vi "19.2-Signal-Generator-FFT.vi"() -> ()   [LabVIEW 2020]
uses:
  <vilib>/Analysis/1siggen.llb/Ramp Pattern by Samples.vi
  <vilib>/Analysis/2dsp.llb/Real FFT.vi
  <vilib>/Analysis/1siggen.llb/General Gauss-Mod Sine.vi
  <vilib>/Analysis/1siggen.llb/General Gaussian Monopulse.vi
  <vilib>/Analysis/1siggen.llb/General Aperiodic Triangle.vi
  <vilib>/Analysis/1siggen.llb/General Periodic Sinc.vi
  <vilib>/Analysis/NI_AALBase.lvlib
  <vilib>/Analysis/NI_AALPro.lvlib
panel:
  in  "Stop":bool
  out "F-Im":dbl[](graph) caption="ImX[k]"
  out "F-Re":dbl[](graph) caption="ReX[k]"
  out "F-Phase":dbl[](graph) caption="PhaseX[k]"
  out "F-Amplitude":dbl[](graph) caption="MagX[k]"
  in  "dt":dbl=0.2
  in  "Delay":i32=50
  in  "SigFrequency":dbl=1.0 format="%.2f"
  in  "Samples":i32=128
  in  "Duration":dbl=1.0 format="%0.2f"
  in  "dc offset":dbl format="%0.2f"
  in  "Phase":dbl format="%0.2f"
  in  "Amplitude":dbl=1.0 format="%.2f"
  in  "Tab":T1(tab)
  in  "Duty (%)":dbl=50.0 format="%0.2f"
  in  "Width":i32=20
  in  "Am/Dm":cluster{"Am":dbl, "Dm":dbl}[](array[cluster])=[{"Am"=5.0, "Dm"=1.0}, {"Am"=3.0, "Dm"=8.0}, {"Am"=1.0, "Dm"=15.0}]
  in  "Interpolation":i32(ring)=1 items=["nearest", "linear", "spline", "cubic Hermite"]
  in  "Pluse":T2(ring)
  in  "delay":dbl=12.0 format="%#_13g"
  in  "f2":dbl=0.1 format="%0.2f"
  in  "f1":dbl=0.01 format="%0.2f"
  in  "Type":u16(ring) items=["Monopulse", "Gaussian Modulated Sine "]
  out "Signal":dbl[](graph)
  out "Error":i32
  out "Phase out":dbl format="%.2f"
  # "Common Parameters"
  # "Signal Generator-FFT"
  # "Instruction:\n1) Select signal from tab;\n2) Set parameters of selected signals;\n3) Run VI and check out the wave and frequency of the signal;\n4) Repeat step 1-3 to see other signal."
  # "Hz"
  # "Move phase of Sine wave 90degrees"
  # "Start=0;\nEnd=A"
  # "Start=A;\nEnd=0"
  # "Add Multi-tones and Gauss white noise"
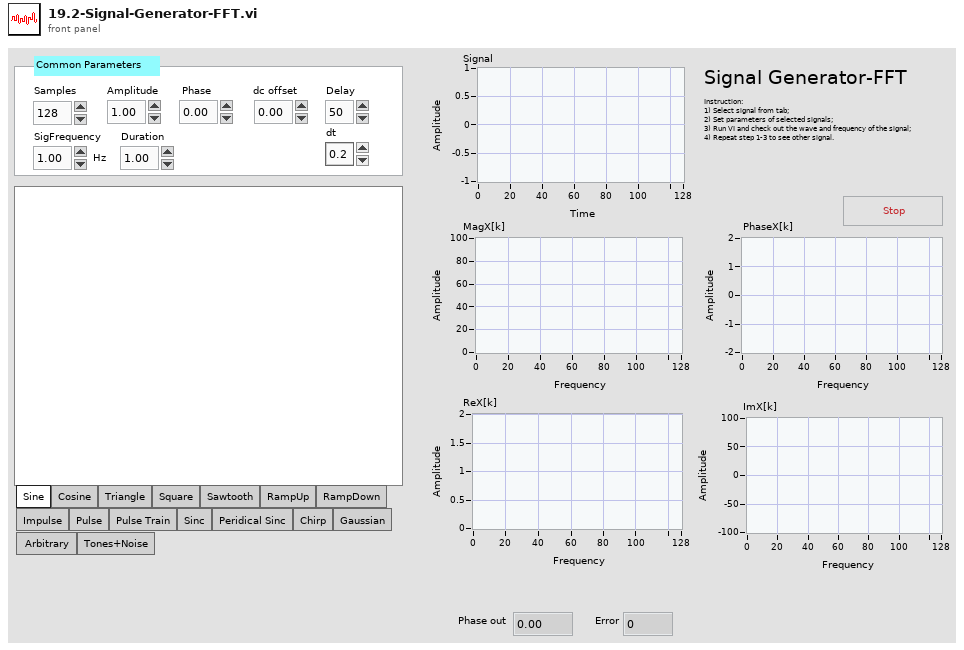
[diagram p1: front panel]
types:
  T1 = enum32{"Sine", "Cosine", "Triangle", "Square", "Sawtooth", "RampUp", "RampDown", "Impulse", "Pulse", "Pulse Train", "Sinc", "Peridical Sinc", "Chirp", "Gaussian", "Arbitrary ", "Tones+Noise"}
  T2 = enum16{"Gauss Mod-Sine", "Gauss Monopulse", "Triangle", "Sine", "Square", "Sinc"}
  T3 = cluster{"frequency":dbl, "amplitude":dbl, "phase":dbl}[]
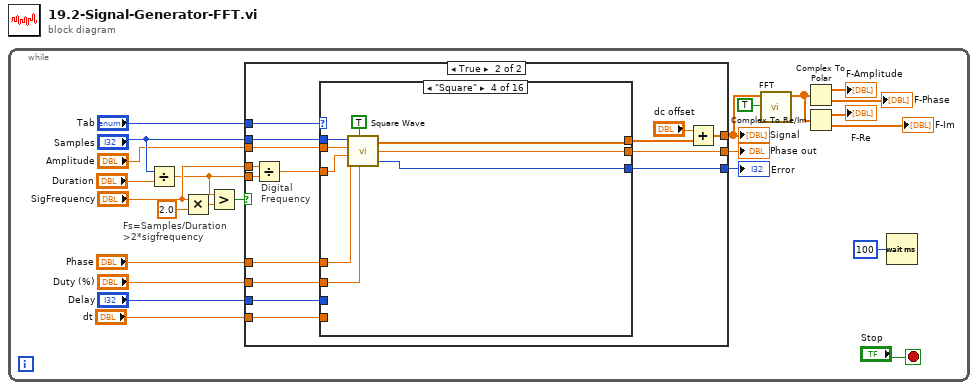
[diagram p0: block diagram]
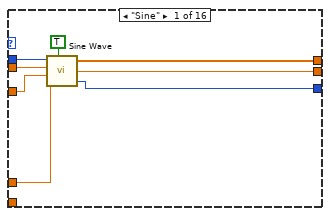
[diagram p3: hidden frame]
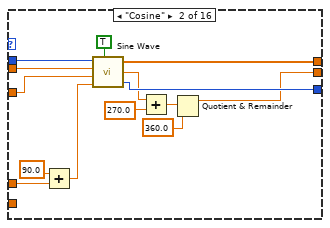
[diagram p4: hidden frame]
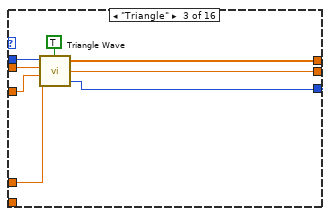
[diagram p5: hidden frame]
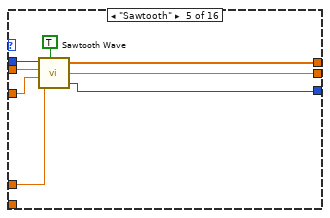
[diagram p6: hidden frame]
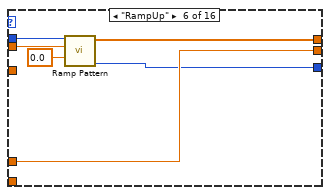
[diagram p7: hidden frame]
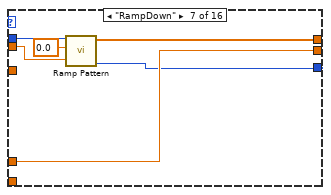
[diagram p8: hidden frame]
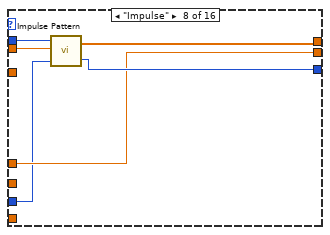
[diagram p9: hidden frame]
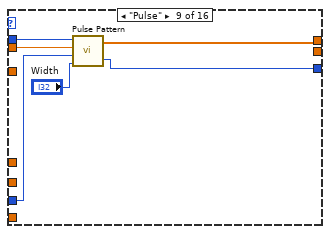
[diagram p10: hidden frame]
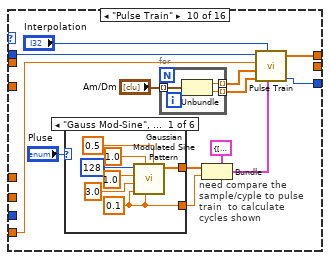
[diagram p11: hidden frame]
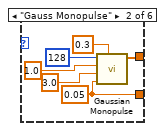
[diagram p12: hidden frame]
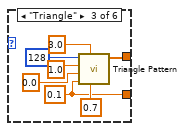
[diagram p13: hidden frame]
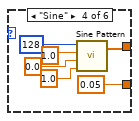
[diagram p14: hidden frame]
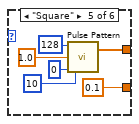
[diagram p15: hidden frame]
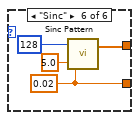
[diagram p16: hidden frame]
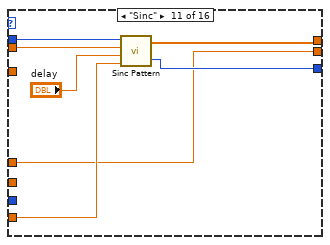
[diagram p17: hidden frame]
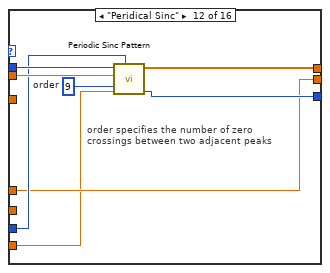
[diagram p18: hidden frame]
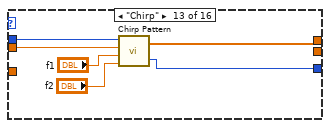
[diagram p19: hidden frame]
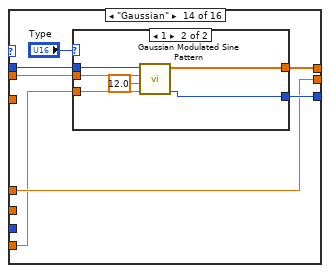
[diagram p20: hidden frame]
diagram:
  n1 = while {
    stop <- "Stop" stop-if-true
    # "Fs=Samples/Duration \n>2*sigfrequency"
    n2 = Divide(x="Samples", y="Duration") -> (x/y=w13:dbl)
    n3 = Multiply(x="SigFrequency", y=2.0) -> (x*y=w12:dbl)
    n4 = Greater?(x=w13, y=w12) -> (0:w16:bool)
    n5 = case shown="True" w16 {
      tunnel: w13 -> [_ w42]
      tunnel: "Samples" -> [_ w41]
      tunnel: "SigFrequency" -> [_ w31]
      tunnel: [-20061 ("error") w37] -> w24
      tunnel: [dbl[] [] ("Signal") w36] -> w9
      tunnel: "Tab" -> [_ w35]
      tunnel: "Amplitude" -> [_ w34]
      tunnel: "Phase" -> [w25 w33]
      tunnel: "Duty (%)" -> [_ w32]
      tunnel: [w25 w30] -> w17
      tunnel: "Delay" -> [_ w29]
      tunnel: "dt" -> [_ w28]
      frame False {
        # "Error: Nyquist Criterion violated\nsamples/duration must be > 2*frequency\nYou must adjust samples, duration, or frequency by:\n     increasing #samples\n     decreasing duration\n     decreasing frequency"
      }
      frame True {
        # "Digital \nFrequency"
        n6 = Divide(x=w31, y=w42) -> (x/y=w40:dbl)
        n7 = case shown="\"Square\"" w35 {
          tunnel: w34 -> [w50 w64 w72 w81 w83 w94 w98 w106 w113 _ w171 w180 w186 w193 w214 _]
          tunnel: w33 -> [w49 w51 w71 w80 w89 w91 w97 w103 _ _ w167 w174 _ w189 w211 _]
          tunnel: [w48 w60 w67 w74 w84 w92 w100 w104 w108 w124 w170 w175 w183 w190 w208 w217] -> w38
          tunnel: w41 -> [w47 w63 w70 w78 w88 w95 w101 w107 w112 w126 w172 w179 w185 w192 w213 w218]
          tunnel: w40 -> [w43 w53 w65 w79 w86 _ _ _ _ _ _ _ _ _ w212 _]
          tunnel: [w46 w55 w69 w77 w87 w91 w97 w103 _ _ w167 w174 _ w189 w209 _] -> w30
          tunnel: w32 -> [_ _ _ w76 _ _ _ _ _ _ _ _ _ _ _ _]
          tunnel: [w45 w59 w66 w73 w82 w90 w96 w105 w109 w125 w169 w176 w184 w191 w210 _] -> w37
          tunnel: w29 -> [_ _ _ _ _ _ _ w102 w111 _ _ w178 _ _ _ _]
          tunnel: w28 -> [_ _ _ _ _ _ _ _ _ w114 w168 w173 _ w188 _ _]
          frame "Sine" {
            n8 = call <vilib>:"Sine Wave.vi"("samples"=w47, "amplitude"=w50, "frequency"=w43, "phase in"=w49, "reset phase"=TRUE) -> ("sine wave"=w48:dbl[], "phase out"=w46:dbl, "error"=w45:i32)
          }
          frame "Cosine" {
            n9 = Add(x=90.0 ("y"), y=w51) -> (x+y=w61:dbl)
            n10 = call <vilib>:"Sine Wave.vi"("samples"=w63, "amplitude"=w64, "frequency"=w53, "phase in"=w61, "reset phase"=TRUE) -> ("sine wave"=w60:dbl[], "phase out"=w57:dbl, "error"=w59:i32)
            n11 = Add(x=w57, y=270.0) -> (x+y=w54:dbl)
            n12 = Quotient & Remainder(x=w54, y=360.0) -> (x-y*floor(x/y)=w55:dbl)  [unwired: 1 out]
          }
          frame "Triangle" {
            n13 = call <vilib>:"Triangle Wave.vi"("samples"=w70, "amplitude"=w72, "frequency"=w65, "phase in"=w71, "reset phase"=TRUE) -> ("triangle wave"=w67:dbl[], "phase out"=w69:dbl, "error"=w66:i32)
          }
          frame "Square" {
            n14 = call <vilib>:"Square Wave.vi"("samples"=w78, "reset phase"=TRUE, "amplitude"=w81, "frequency"=w79, "duty cycle (%)"=w76, "phase in"=w80) -> ("square wave"=w74:dbl[], "phase out"=w77:dbl, "error"=w73:i32)
          }
          frame "Sawtooth" {
            n15 = call <vilib>:"Sawtooth Wave.vi"("samples"=w88, "amplitude"=w83, "frequency"=w86, "phase in"=w89, "reset phase"=TRUE) -> ("sawtooth wave"=w84:dbl[], "phase out"=w87:dbl, "error"=w82:i32)
          }
          frame "RampUp" {
            n16 = call-poly <vilib>:"Ramp Pattern.vi"("start"=0.0, "end"=w94, "samples"=w95) -> ("error"=w90:i32, "Ramp Pattern"=w92:dbl[])  [unwired: 7 in]
          }
          frame "RampDown" {
            n17 = call-poly <vilib>:"Ramp Pattern.vi"("start"=w98, "end"=0.0 ("start"), "samples"=w101) -> ("error"=w96:i32, "Ramp Pattern"=w100:dbl[])  [unwired: 7 in]
          }
          frame "Impulse" {
            n18 = call <vilib>:"Impulse Pattern.vi"("delay"=w102, "amplitude"=w106, "samples"=w107) -> ("error"=w105:i32, "Impulse Pattern"=w104:dbl[])
          }
          frame "Pulse" {
            n19 = call <vilib>:"Pulse Pattern.vi"("width"="Width", "delay"=w111, "amplitude"=w113, "samples"=w112) -> ("error"=w109:i32, "Pulse Pattern"=w108:dbl[])
          }
          frame "Pulse Train" {
            # "need compare the sample/cyple to pulse train  to calculate cycles shown"
            n20 = case shown="\"Gauss Mod-Sine\", Default" "Pluse" {
              tunnel: [w133 w139 w143 w148 w158 w161] -> w115
              tunnel: [w127 w134 w142 0.05 0.1 ("delta t") w160] -> w118
              frame "Gauss Mod-Sine", Default {
                w127 = 0.1
                n21 = call <vilib>:"Gaussian Modulated Sine Pattern.vi"("attenuation (dB)"=0.5 ("attenuation"), "normalized bandwidth"=w127, "center frequency (Hz)"=1.0 ("center frequency"), "delta t (s)"=w127, "delay (s)"=3.0 ("delay"), "amplitude"=1.0, "samples"=128) -> ("Gauss-Mod Sine Pattern"=w133:dbl[])  [unwired: 3 in, 1 out]
              }
              frame "Gauss Monopulse" {
                w134 = 0.05 ("delta t")
                n22 = call <vilib>:"Gaussian Monopulse.vi"("center frequency (Hz)"=0.3 ("center frequency"), "delta t (s)"=w134, "delay (s)"=3.0 ("delay"), "amplitude"=1.0, "samples"=128) -> ("Gaussian Monopulse"=w139:dbl[])  [unwired: 5 in, 1 out]
              }
              frame "Triangle" {
                w142 = 0.1 ("delta t")
                n23 = call <vilib>:"Triangle Pattern.vi"("asymmetry"=0.7, "width (s)"=3.0 ("width"), "delta t (s)"=w142, "delay (s)"=0.0 ("delay"), "amplitude"=1.0, "samples"=128) -> ("Triangle Pattern"=w143:dbl[])  [unwired: 4 in, 1 out]
              }
              frame "Sine" {
                n24 = call <vilib>:"Sine Pattern.vi"("cycles"=1.0, "phase(degrees)"=0.0, "amplitude"=1.0, "samples"=128 ("samples 2")) -> ("Sinusoidal Pattern"=w148:dbl[])  [unwired: 1 out]
              }
              frame "Square" {
                n25 = call <vilib>:"Pulse Pattern.vi"("width"=10, "delay"=0, "amplitude"=1.0, "samples"=128) -> ("Pulse Pattern"=w158:dbl[])  [unwired: 1 out]
              }
              frame "Sinc" {
                w160 = 0.02 ("delta t")
                n26 = call <vilib>:"Sinc Pattern.vi"("delta t"=w160, "delay"=5.0, "samples"=128) -> ("Sinc Pattern"=w161:dbl[])  [unwired: 1 in, 1 out]
              }
            }
            n27 = for {
              tunnel: "Am/Dm" -> [w165] mode=indexing
              tunnel: [w164] -> w121 mode=indexing
              tunnel: [w163] -> w120 mode=indexing
              n28 = Unbundle(w165) -> ("Am"=w164:dbl, "Dm"=w163:dbl)
            }
            n29 = Bundle(cluster=cluster{"Sinusoidal Pattern":dbl[], dbl} {"Sinusoidal Pattern"=[], 0.0} ("output cluster"), "Sinusoidal Pattern"=w115, w118) -> (w117:cluster{"Sinusoidal Pattern":dbl[], dbl})
            n30 = call <vilib>:"Pulse Train.vi"("prototype spec"=w117, "interpolation method"="Interpolation", "Delay (s)"=w120, "Amplitude"=w121, "delta t of pulse train (s)"=w114, "samples"=w126) -> ("error"=w125:i32, "Pulse Train"=w124:dbl[])  [unwired: 4 in]
          }
          frame "Sinc" {
            n31 = call <vilib>:"Sinc Pattern.vi"("delta t"=w168, "delay"="delay", "amplitude"=w171, "samples"=w172) -> ("error"=w169:i32, "Sinc Pattern"=w170:dbl[])
          }
          frame "Peridical Sinc" {
            w177 = 9  # order
            # "order specifies the number of zero \ncrossings between two adjacent peaks"
            n32 = call <vilib>:"Periodic Sinc Pattern.vi"("delay (s)"=w178, "delta t (s)"=w173, "order"=w177, "amplitude"=w180, "samples"=w179) -> ("error"=w176:i32, "Periodic Sinc Pattern"=w175:dbl[])  [unwired: 5 in]
          }
          frame "Chirp" {
            n33 = call <vilib>:"Chirp Pattern.vi"("f2"="f2", "f1"="f1", "amplitude"=w186, "samples"=w185) -> ("error"=w184:i32, "Chirp Pattern"=w183:dbl[])
          }
          frame "Gaussian" {
            n34 = case shown="1" "Type" {
              tunnel: w193 -> [w199 w203]
              tunnel: w192 -> [w198 w204]
              tunnel: [w197 w202] -> w191
              tunnel: [w196 w201] -> w190
              tunnel: w188 -> [w195 w205]
              frame 0, Default {
                n35 = call <vilib>:"Gaussian Monopulse.vi"("delta t (s)"=w195, "delay (s)"=12.0, "amplitude"=w199, "samples"=w198) -> ("error"=w197:i32, "Gaussian Monopulse"=w196:dbl[])  [unwired: 6 in]
              }
              frame 1 {
                n36 = call <vilib>:"Gaussian Modulated Sine Pattern.vi"("delta t (s)"=w205, "delay (s)"=12.0, "amplitude"=w203, "samples"=w204) -> ("error"=w202:i32, "Gauss-Mod Sine Pattern"=w201:dbl[])  [unwired: 6 in]
              }
            }
          }
          frame "Arbitrary " {
            w206 = 1 items=["none", "linear"]  # interpolation
            w207 = dbl[] [0.0, 1.0, 4.0, 1.0, 8.0, 6.0, 2.0, 1.0]  # Wave Table
            n37 = call <vilib>:"Arbitrary Wave.vi"("interpolation"=w206, "Wave Table"=w207, "phase in"=w211, "frequency"=w212, "amplitude"=w214, "samples"=w213) -> ("error"=w210:i32, "phase out"=w209:dbl, "arbitrary wave"=w208:dbl[])  [unwired: 1 in]
          }
          frame "Tones+Noise" {
            n38 = call <vilib>:"Tones and Noise.vi"("noise (rms)"=0.1, "tones"=T3 [{"frequency"=10.0, "amplitude"=5.0, "phase"=0.0}, {"frequency"=20.0, "amplitude"=0.1, "phase"=0.0}, {"frequency"=40.0, "amplitude"=1.0, "phase"=0.0}, {"frequency"=600.0, "amplitude"=2.0, "phase"=0.0}], "samples"=w218) -> ("tones and noise"=w217:dbl[])  [unwired: 7 in, 1 out]
          }
        }
        n39 = Add(x="dc offset", y=w38) -> (x+y=w36:dbl[])
      }
    }
    "Error" <- w24
    "Signal" <- w9
    "Phase out" <- w17
    n40 = call-poly <vilib>:"FFT.vi"("shift?"=TRUE, "X"=w9) -> ("FFT {X}"=w6:cdb[])  [unwired: 8 in, 1 out]
    n41 = Complex To Polar(r * e^(i*theta)=w6) -> (r=→"F-Amplitude":dbl[], theta=→"F-Phase":dbl[])
    n42 = Complex To Re/Im(x + iy=w6) -> (x=→"F-Re":dbl[], y=→"F-Im":dbl[])
    n43 = Wait (ms)(milliseconds to wait=u32 100) -> ()  [unwired: 1 out]
  }
